vi "GUI Wavefrom Panel.vi"(8 "error in":errorcluster, 11 "source name":string="last record") -> (0 "error out":errorcluster)   [LabVIEW 2018]
doc: "Viewer of the record waveforms."
uses:
  GUI Waveform Info.ctl
panel:
  in  "avg index":u16(ring) caption="Average index" items=["Last", "Cycle 1"]
  in  "grp index":u16(ring) caption="Group index" items=["Last", "Group 1"]
  in  "max smpl":i32=1000 caption="Max samples to display"
  out "Channel waveforms":T1(graph)
  out "Current record path":path
  in  "first smpl [%]":dbl(slide) caption="First sample to display [%]" min=0.0 max=100.0 step=0.1 scale=0.0..100.0
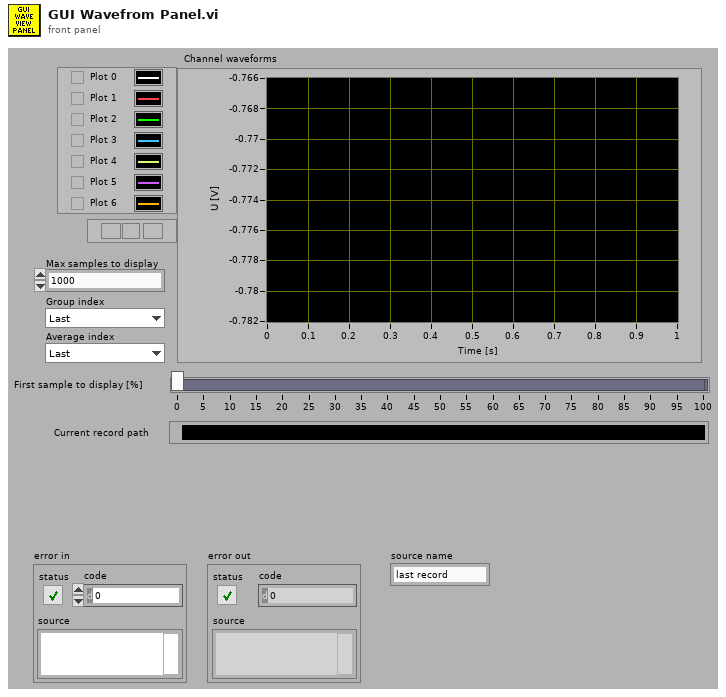
[diagram p1: front panel]
types:
  T1 = cluster{"time [s]":ext[], "waveforms [V]":sgl[]}[]
  T2 = typedef "GUI Waveform Info.ctl" = cluster{"header path":path, "group id":i32, "average id":i32, "Time Stamp":timestamp, "max samples":i64, "first sample":i64, "first smpl [%]":dbl, "kill viewer":bool}
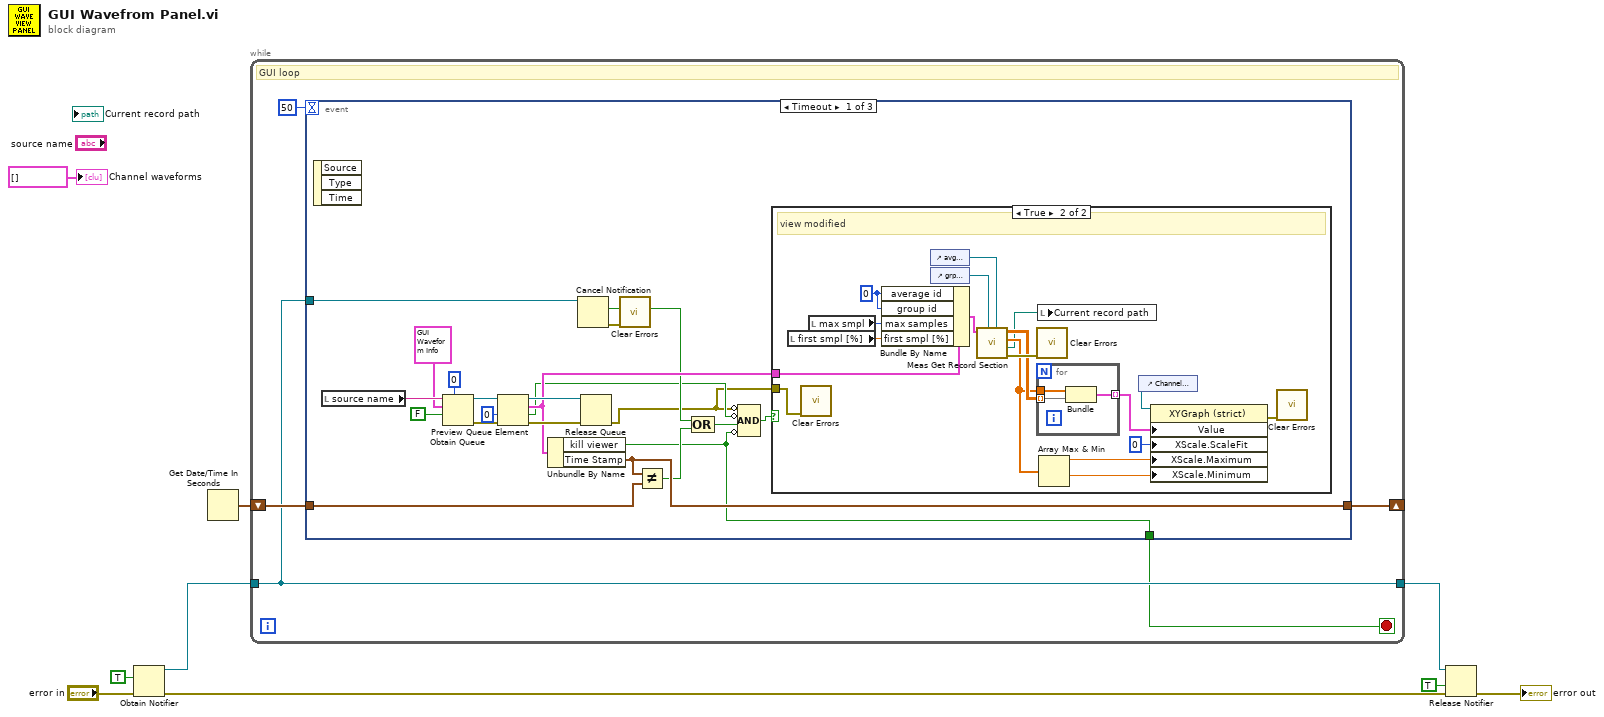
[diagram p0: block diagram]
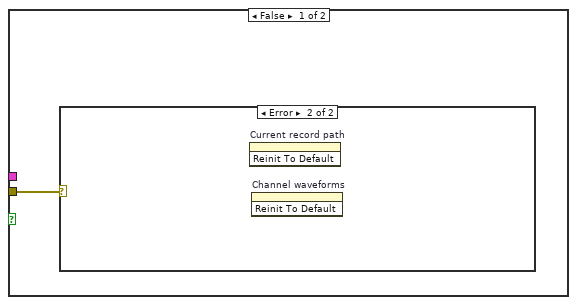
[diagram p2: hidden frame]
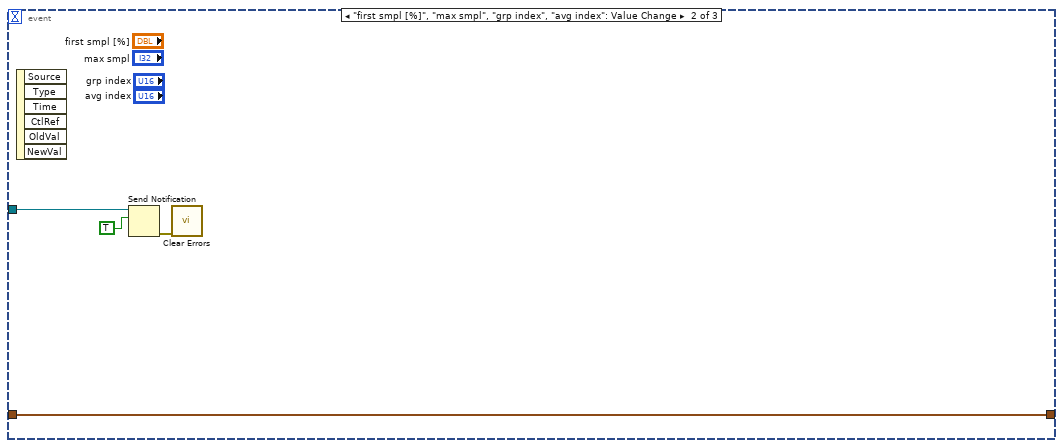
[diagram p4: hidden frame]
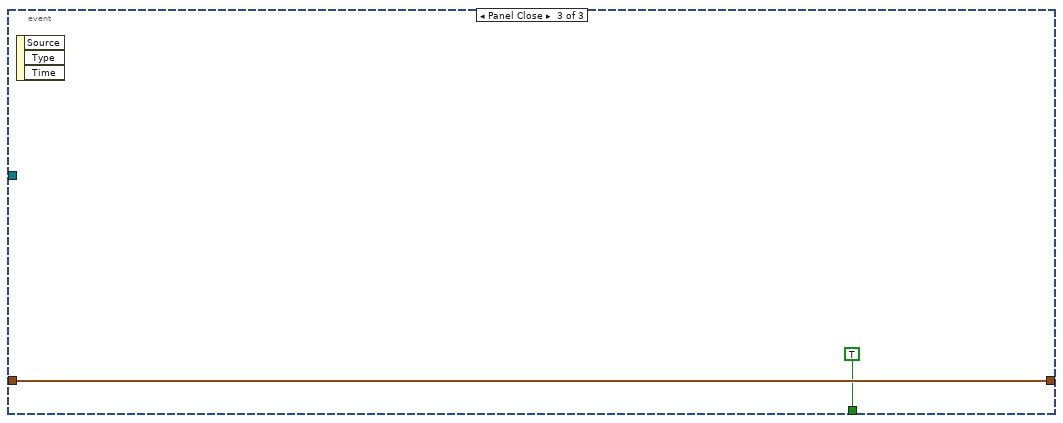
[diagram p5: hidden frame]
diagram:
  n1 = Obtain Notifier(notification data type=TRUE, error in (no error)="error in") -> (notifier out=w2:refnum<notifier>, error out=w6:errorcluster)  [unwired: 2 in, 1 out]
  n2 = Get Date/Time In Seconds() -> (seconds since 1Jan1904=w9:timestamp)
  n3 = while {
    shift-right: [w12] -> _
    shift-left: w9 -> [w13]
    tunnel: [w11] -> w3
    tunnel: w2 -> [w11]
    stop <- w10 stop-if-true
    # "GUI loop"
    n4 = event shown="[0] Timeout" {
      selector: _ -> [_ _ _]
      dyn-events: _ -> [_ _ _]
      timeout: 50 -> [_ _ _]
      tunnel: w13 -> [w27 w61 w63]
      tunnel: [w26 w61 w63] -> w12
      tunnel: w11 -> [w24 w60 _]
      tunnel: [w15 _ TRUE] -> w10
      event Timeout {
        n5 = event-data() -> ()  [unwired: 1 in, 3 out]
        n6 = local read "source name"() -> (w35:string)
        n7 = Obtain Queue(max queue size (-1, unlimited)=0, name (unnamed)=w35, element data type=T2 {"header path"=path "", "group id"=0, "average id"=0, "Time Stamp"=timestamp(0 s since 1904-01-01), "max samples"=0, "first sample"=0, "first smpl [%]"=0.0, "kill viewer"=FALSE} ("record info"), create if not found? (T)=FALSE) -> (queue out=w32:refnum<queue>, error out=w17:errorcluster)  [unwired: 1 in, 1 out]
        n8 = Preview Queue Element(queue=w32, timeout in ms (-1)=0, error in (no error)=w17) -> (queue out=w31:refnum<queue>, element=w25:T2, timed out?=w18:bool, error out=w33:errorcluster)
        n9 = Unbundle By Name(w25) -> ("kill viewer"=w15:bool, "Time Stamp"=w26:timestamp)
        n10 = Cancel Notification(0:w24) -> (9:w22:bool, 11:w21:errorcluster)  [unwired: 1 in, 1 out]
        n11 = Release Queue(queue=w31, error in (no error)=w33) -> (error out=w16:errorcluster)  [unwired: 1 in, 2 out]
        n12 = call <vilib>:"Clear Errors.vi"("error in (no error)"=w21) -> ()  [unwired: 5 in, 2 out]
        n13 = Not Equal?(x=w26, y=w27) -> (x != y?=w23:bool)
        n14 = Compound Arithmetic op=OR(w22, w23) -> (w20:bool)
        n15 = Compound Arithmetic op=AND(invert w16, invert w18, w20, invert w15) -> (w19:bool)
        n16 = case shown="True" w19 {
          tunnel: w25 -> [_ w54]
          tunnel: w16 -> [w36 w37]
          frame False {
            n17 = case shown="Error" w36 {
              frame No Error {
              }
              frame Error {
                n18 = invoke on="Current record path" class="Path" method="Reinit To Default"() -> ()  [unwired: 3 in, 3 out]
                n19 = invoke on="Channel waveforms" class="XYGraph (strict)" method="Reinit To Default"() -> ()  [unwired: 3 in, 3 out]
              }
            }
          }
          frame True {
            w40 = 0 ("average id")
            # "view modified"
            n20 = local read "first smpl [%]"() -> (w52:dbl)
            n21 = call <vilib>:"Clear Errors.vi"("error in (no error)"=w37) -> ()  [unwired: 5 in, 2 out]
            n22 = local read "max smpl"() -> (w53:i32)
            n23 = Bundle By Name(cluster=w54, "average id"=w40, "group id"=w40, "max samples"=w53, "first smpl [%]"=w52) -> (w51:T2)
            n24 = control-ref of="avg index"() -> (w38:refnum<vi>)
            n25 = control-ref of="grp index"() -> (w39:refnum<vi>)
            n26 = call "Meas Get Record Section.vi"("avg index ref"=w38, "grp index ref"=w39, "record info"=w51) -> ("error out"=w50:errorcluster, "record path"=w41:path, "time [s]"=w47:ext[], "waveforms [V]"=w49:sgl[][])  [unwired: 5 in]
            n27 = call <vilib>:"Clear Errors.vi"("error in (no error)"=w50) -> ()  [unwired: 5 in, 2 out]
            n28 = for {
              tunnel: w49 -> [w57] mode=indexing
              tunnel: w47 -> [w56]
              tunnel: [w55] -> w43 mode=indexing
              n29 = Bundle("time [s]"=w56, "waveforms [V]"=w57) -> (w55:cluster{"time [s]":ext[], "waveforms [V]":sgl[]})  [unwired: 1 in]
            }
            n30 = local write "Current record path"(w41) -> ()
            n31 = Array Max & Min(array=w47) -> (max value=w46:ext, min value=w45:ext)  [unwired: 2 out]
            n32 = control-ref of="Channel waveforms"() -> (w48:refnum<vi>)
            n33 = property class="XYGraph (strict)"(reference=w48, "Value"=w43, "XScale.ScaleFit"=u8 0 ("X Scale.Scale Fit"), "XScale.Maximum"=w46, "XScale.Minimum"=w45) -> (error out=w44:errorcluster)  [unwired: 1 in, 1 out]
            n34 = call <vilib>:"Clear Errors.vi"("error in (no error)"=w44) -> ()  [unwired: 5 in, 2 out]
          }
        }
      }
      event "first smpl [%]", "max smpl", "grp index", "avg index": Value Change {
        n35 = event-data() -> ()  [unwired: 1 in, 6 out]
        n36 = Send Notification(notification=TRUE, notifier=w60) -> (error out=w58:errorcluster)  [unwired: 1 in, 1 out]
        n37 = call <vilib>:"Clear Errors.vi"("error in (no error)"=w58) -> ()  [unwired: 5 in, 2 out]
      }
      event Panel Close {
        n38 = event-data() -> ()  [unwired: 1 in, 3 out]
      }
    }
  }
  n39 = Release Notifier(notifier=w3, force destroy? (F)=TRUE, error in (no error)=w6) -> (error out=→"error out":errorcluster)  [unwired: 2 out]
  "Channel waveforms" <- T1 [] ("XY Graph")
